vi "getTopicName.vi"(8 "error in (no error)":errorcluster, 11 "PUBLISH in":refnum<class "PUBLISH.lvclass">) -> (0 "error out":errorcluster, 2 "Topic":string, 3 "PUBLISH out":refnum<class "PUBLISH.lvclass">)   [LabVIEW 2013, in "PUBLISH.lvclass"]
uses:
  PUBLISH.lvclass
  ControlPacket/ControlPacket.lvclass/ControlPacket.ctl
  ControlPacket/ControlPacket.lvclass
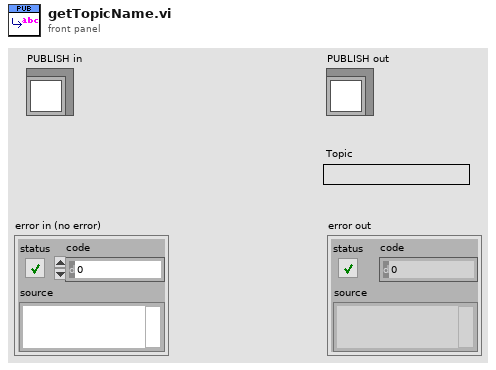
[diagram p1: front panel]
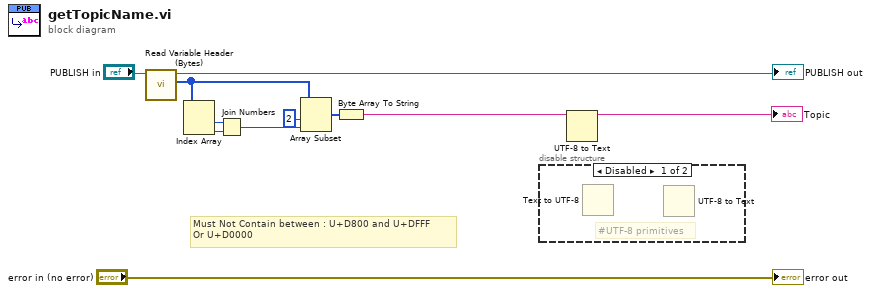
[diagram p0: block diagram]
diagram:
  # "Must Not Contain between : U+D800 and U+DFFF\nOr U+D0000"
  n1 = call "Read Variable Header (Bytes).vi"("ControlPacket in"="PUBLISH in") -> ("Variable Header (Bytes)"=w6:u8[], "ControlPacket out"=→"PUBLISH out":refnum<class "PUBLISH.lvclass">)  [unwired: 9 in]
  n2 = Index Array(array=w6) -> (element #1=w8:u8, element #2=w9:u8)  [unwired: 2 in]
  n3 = Join Numbers(hi=w8, lo=w9) -> ((hi.lo)=w1:u16)
  n4 = Array Subset(array=w6, index=2, length=w1) -> (w7:u8[])
  n5 = Byte Array To String(unsigned byte array=w7) -> (string=w3:string)
  n6 = disable-structure shown="Disabled" {
    frame Disabled {
      # "#UTF-8 primitives"
      n7 = Text to UTF-8() -> ()  [unwired: 2 in, 2 out]
      n8 = UTF-8 to Text() -> ()  [unwired: 2 in, 2 out]
    }
    frame Enabled {
    }
  }
  n9 = UTF-8 to Text(11:w3) -> (3:→"Topic":string)  [unwired: 1 in, 1 out]
  "error out" <- "error in (no error)"
